vi "Actor Core.vi"(8 "error in":errorcluster, 11 "Nested in":refnum<class "BPG.lvclass">) -> (0 "error out":errorcluster, 3 "Actor out":refnum<class "Actor.lvclass">)   [LabVIEW 2021, in "BPG.lvclass"]
doc: "(<B>Filename</B>: Actor Framework.lvlib:Actor.lvclass:Actor Core.vi)\n\nReceives messages to the actor, reacts to them, and initiates any error handling that may shut the actor down.\n\nDescendant classes may override this VI to append parallel tasks for the actor to complete while it handles messages. Overrides use the Call Parent Method node."
uses:
  BPG.lvclass
  C:/Program Files/National Instruments/LabVIEW 2021/vi.lib/ActorFramework/Actor/Actor.lvclass
  <vilib>/ActorFramework/Actor/Actor.lvclass
  BPG.lvclass/BPG.ctl
  <vilib>/ActorFramework/Actor/Actor.lvclass/Actor.ctl
  <vilib>/ActorFramework/Message Enqueuer/Message Enqueuer.lvclass/Message Enqueuer.ctl
  <vilib>/ActorFramework/Message Enqueuer/Init from Existing Queue.vi
  <vilib>/ActorFramework/Message Enqueuer/Enqueue.vi
  <vilib>/ActorFramework/Stop Msg/Stop Msg.lvclass
  C:/Program Files/National Instruments/LabVIEW 2021/vi.lib/ActorFramework/Message/Message.lvclass
  <vilib>/ActorFramework/Message Priority Queue/Priority Enqueue.vi
  <vilib>/MGI/Panel Manager/Panel Actor/Panel Actor/Panel Actor.lvclass
  <vilib>/ActorFramework/Message Enqueuer/Message Enqueuer.lvclass
panel:
  out "Status":string
  out "BPG Waveform":waveform(dbl)(graph)
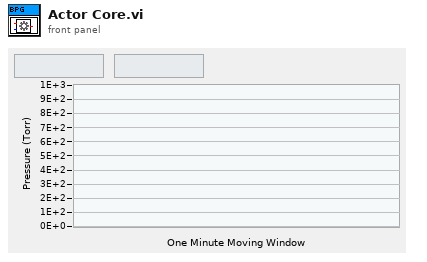
[diagram p1: front panel]
types:
  T1 = cluster{"Stop":refnum<user-event>, "BPG Waveform":refnum<user-event>, "Status":refnum<user-event>}
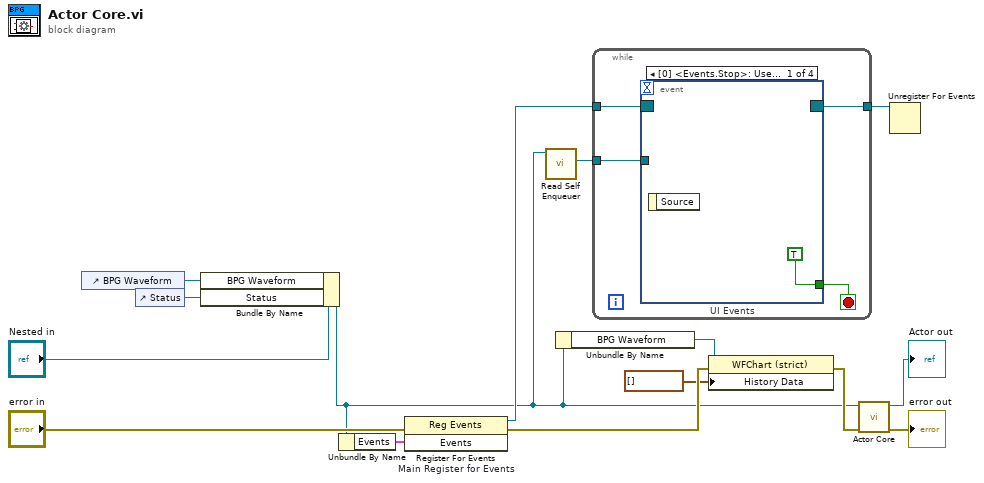
[diagram p0: block diagram]
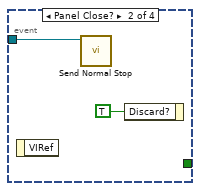
[diagram p2: hidden frame]
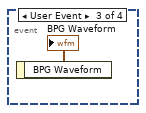
[diagram p3: hidden frame]
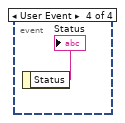
[diagram p4: hidden frame]
diagram:
  n1 = control-ref of="BPG Waveform"() -> (w7:refnum<vi>)
  n2 = control-ref of="Status"() -> (w9:refnum<vi>)
  n3 = Bundle By Name(cluster="Nested in", "BPG Waveform"=w7, "Status"=w9) -> (w1:refnum<class "BPG.lvclass">)
  n4 = Unbundle By Name(w1) -> ("Events"=w12:T1)
  n5 = register-events "Main Register for Events"(error in="error in", w12) -> (reference out=w13:refnum<event-registration>, error out=w4:errorcluster)  [unwired: 1 in]
  n6 = call <vilib>:"Read Self Enqueuer.vi"("Actor"=w1) -> ("Self Enqueuer"=w6:refnum<class "Message Enqueuer.lvclass">)  [unwired: 10 in]
  n7 = Unbundle By Name(w1) -> ("BPG Waveform"=w5:refnum<vi>)
  n8 = while {
    tunnel: w13 -> [w19]
    tunnel: [w17] -> w11
    tunnel: w6 -> [w16]
    stop <- w18 stop-if-true
    n9 = event "UI Events" shown="[0] <Events.Stop>: User Event" {
      selector: w19 -> [_ _ _ _]
      dyn-events: [_ _ _ _] -> w17
      timeout: _ -> [_ _ _ _]
      tunnel: [TRUE _ _ _] -> w18
      tunnel: w16 -> [_ w21 _ _]
      event User Event {
        n10 = event-data() -> ()  [unwired: 1 in, 1 out]
      }
      event Panel Close? {
        n11 = event-data() -> ()  [unwired: 1 in, 1 out]
        n12 = call <vilib>:"Send Normal Stop.vi"("Message Enqueuer"=w21) -> ()  [unwired: 10 in, 1 out]
        n13 = event-data("Discard?"=TRUE) -> ()  [unwired: 1 in, 1 out]
      }
      event User Event {
        n14 = event-data() -> ("BPG Waveform"=→"BPG Waveform":waveform(dbl))  [unwired: 1 in]
      }
      event User Event {
        n15 = event-data() -> ("Status"=→"Status":string)  [unwired: 1 in]
      }
    }
  }
  n16 = property class="WFChart (strict)"(reference=w5, error in=w4, "History Data"=waveform(dbl)[] []) -> (error out=w3:errorcluster)  [unwired: 1 out]
  n17 = call-parent "Actor Core.vi"("error in"=w3, "Panel Actor in"=w1) -> ("error out"=→"error out":errorcluster, "Actor out"=→"Actor out":refnum<class "Actor.lvclass">)  [unwired: 8 in]
  n18 = Unregister For Events(event registration refnum=w11) -> ()  [unwired: 1 in, 1 out]
